vi "Create Command.vi"(10 "Path to file":path) -> (3 "Load.lvclass":refnum<class "Load.lvclass">)   [LabVIEW 2010, in "Load.lvclass"]
doc: "This instance of Create Command.vi writes the value of the Path to file input to the data stored within Load.lvclass."
uses:
  Load.lvclass
  Load.lvclass/Load.ctl
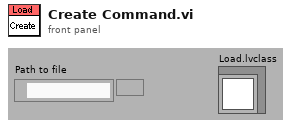
[diagram p1: front panel]
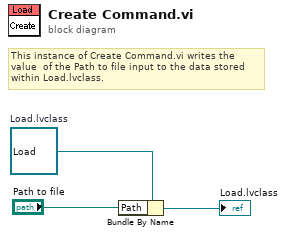
[diagram p0: block diagram]
diagram:
  w3 = refnum<class "Load.lvclass"> refnum  # Load.lvclass
  # "This instance of Create Command.vi writes the value  of the Path to file input to the data stored within Load.lvclass."
  n1 = Bundle By Name "Bundle By Name"(cluster=w3, "Path"="Path to file") -> (→"Load.lvclass":refnum<class "Load.lvclass">)
